vi "Set timeline cursors X position.vi"(8 "error in (no error)":errorcluster, 9 "Right":dbl, 10 "Left":dbl, 11 "Timeline Graph in":T1) -> (0 "error out":errorcluster, 3 "Timeline Graph out":T1)   [LabVIEW 2020, in "XGrapher.xctl"]
uses:
  XGrapher.xctl
  Typedefs/Xctrl-Timeline graph ref.ctl
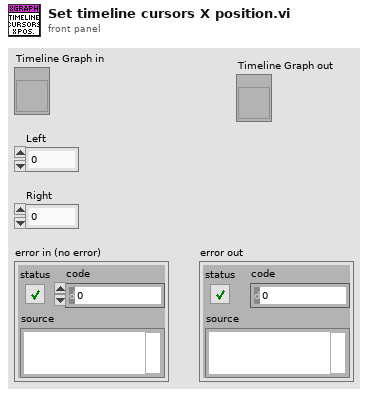
[diagram p1: front panel]
types:
  T1 = typedef "XGrapher.xctl/Xctrl-Timeline graph ref.ctl" = refnum<vi>
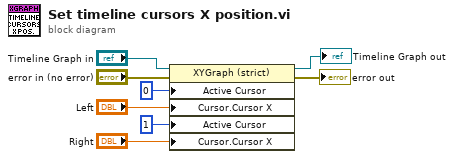
[diagram p0: block diagram]
diagram:
  n1 = property on="Property Node" class="XYGraph (strict)"(reference="Timeline Graph in", error in="error in (no error)", "Active Cursor"=u32 0, "Cursor.Cursor X"="Left", "Active Cursor"=u32 1, "Cursor.Cursor X"="Right") -> (reference out=→"Timeline Graph out":T1, error out=→"error out":errorcluster)
